vi "Move XYZ.vi"(0 "PID Gains In":T2={"X PID"={"proportional gain (Kc)"=0.03, "integral time (Ti, min)"=0.0, "derivative time (Td, min)"=0.0}, "Y PID"={"proportional gain (Kc)"=0.03, "integral time (Ti, min)"=0.0, "derivative time (Td, min)"=0.0}, "Z PID"={"proportional gain (Kc)"=0.035, "integral time (Ti, min)"=0.0, "derivative time (Td, min)"=0.0}} {"Z PID"."derivative time (Td, min)" format="%.3f"; "Z PID"."integral time (Ti, min)" format="%.3f"; "Z PID"."proportional gain (Kc)" format="%.3f"; "Y PID"."derivative time (Td, min)" format="%.3f"; "Y PID"."integral time (Ti, min)" format="%.3f"; "Y PID"."proportional gain (Kc)" format="%.3f"; "X PID"."derivative time (Td, min)" format="%.3f"; "X PID"."integral time (Ti, min)" format="%.3f"; "X PID"."proportional gain (Kc)" format="%.3f"}, 5 "Y Target":dbl, 6 "X Target":dbl, 10 "Max Time":dbl=90.0, 11 "Gyro Target":dbl=-180.0, 12 "Movement":dbl=3.0, 14 "X Output Range":cluster{"output high":dbl, "output low":dbl}={"output high"=0.8, "output low"=-0.8}, 15 "X Stop Threshold":dbl=5.0, 16 "Y Output Range":cluster{"output high":dbl, "output low":dbl}={"output high"=0.8, "output low"=-0.8}, 17 "Y Stop Threshold":dbl=5.0, 18 "Z Output Range":cluster{"output high":dbl, "output low":dbl}={"output high"=0.8, "output low"=-0.8}, 19 "Z  Stop Threshold":dbl=8.0) -> ()   [LabVIEW 2018]
uses:
  Robot Global Data.vi
  SubSystems/Drive Train/Drive Train Global.vi
  SubSystems/Hatch Panel Intake/Hatch Panel Intake Global.vi
  SubSystems/Lift/Lift Global.vi
  <vilib>/addons/control/pid/pid.llb/PID (DBL).vi
  <vilib>/addons/control/pid/NI_PID_pid.lvlib
panel:
  in  "Camera Tracking":T1={"proportional gain (Kc)"=0.06, "integral time (Ti, min)"=0.0, "derivative time (Td, min)"=0.0}
  in  "Minimum Time":u32=500
  in  "Settle Time":u32=2000
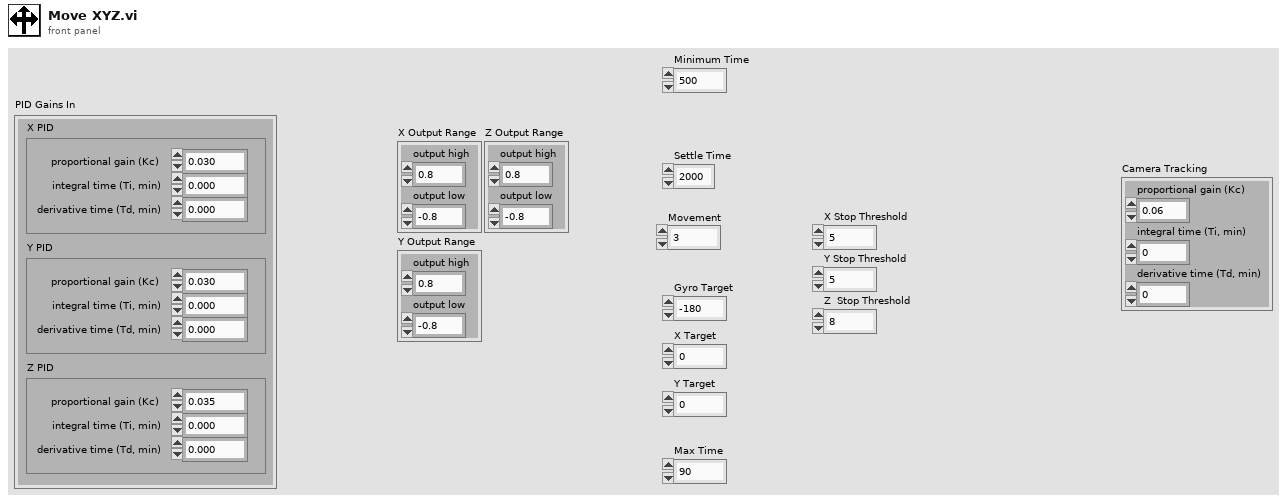
[diagram p1: front panel]
types:
  T1 = cluster{"proportional gain (Kc)":dbl, "integral time (Ti, min)":dbl, "derivative time (Td, min)":dbl}
  T2 = cluster{"X PID":cluster{"proportional gain (Kc)":dbl, "integral time (Ti, min)":dbl, "derivative time (Td, min)":dbl}, "Y PID":cluster{"proportional gain (Kc)":dbl, "integral time (Ti, min)":dbl, "derivative time (Td, min)":dbl}, "Z PID":cluster{"proportional gain (Kc)":dbl, "integral time (Ti, min)":dbl, "derivative time (Td, min)":dbl}}
  T3 = cluster{"Rollover":dbl, "Yaw":dbl, "Cont Yaw":dbl}
  T4 = cluster{"offsetAngle H":dbl, "offsetAngle V":dbl, "area":dbl, "skew":dbl, "validTarget":dbl, "latency":dbl}
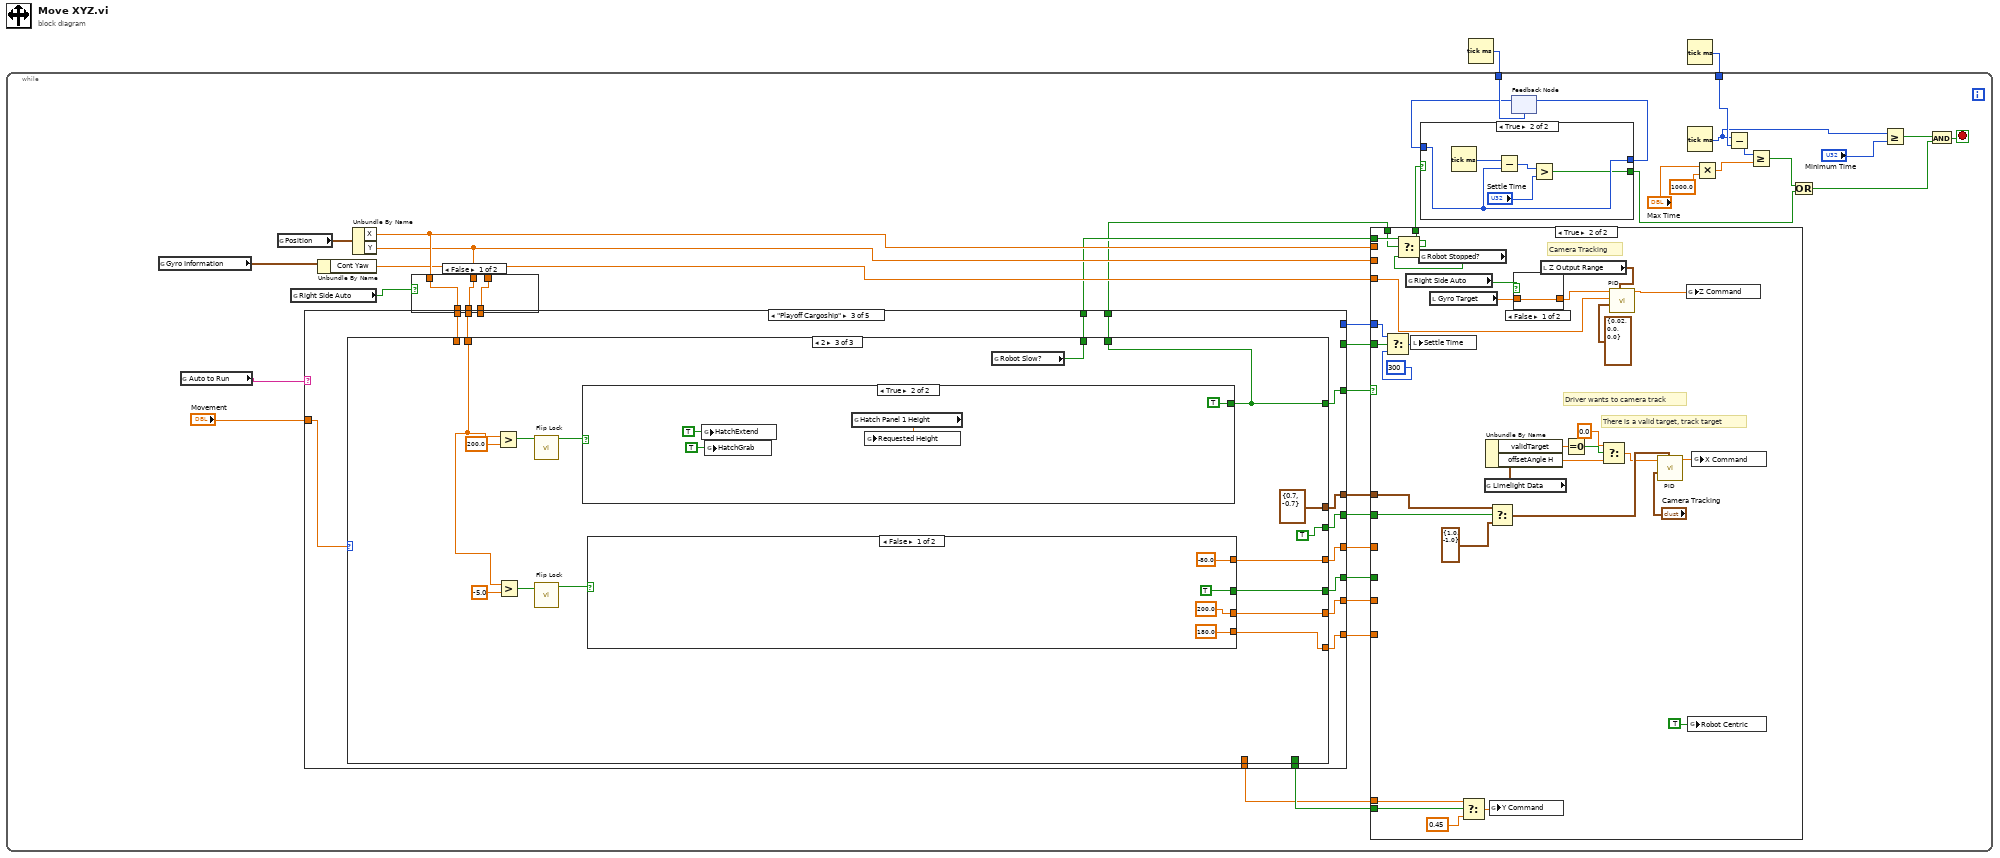
[diagram p0: block diagram]
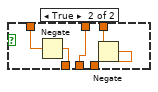
[diagram p2: hidden frame]
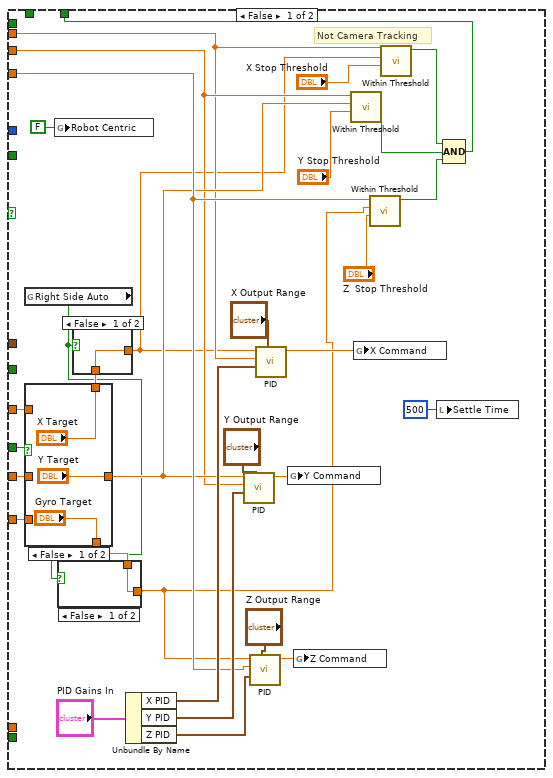
[diagram p3: hidden frame]
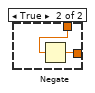
[diagram p4: hidden frame]
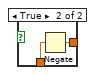
[diagram p5: hidden frame]
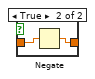
[diagram p7: hidden frame]
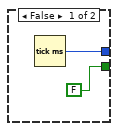
[diagram p8: hidden frame]
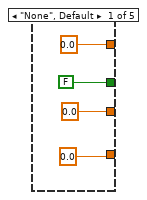
[diagram p9: hidden frame]
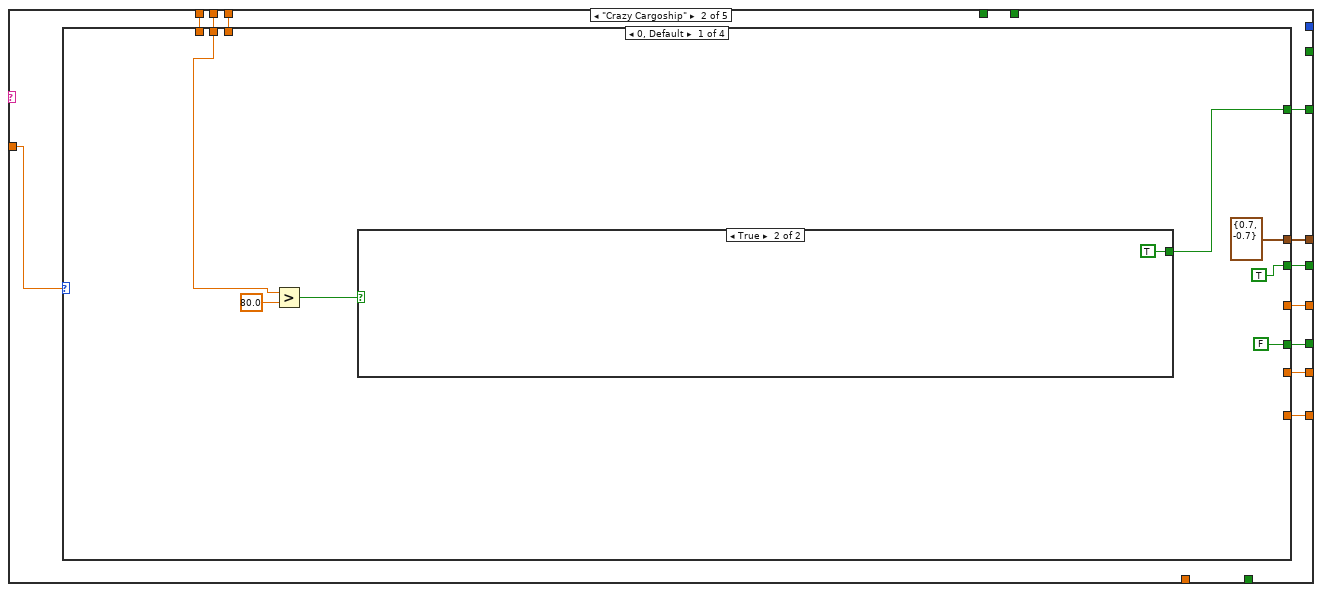
[diagram p10: hidden frame]
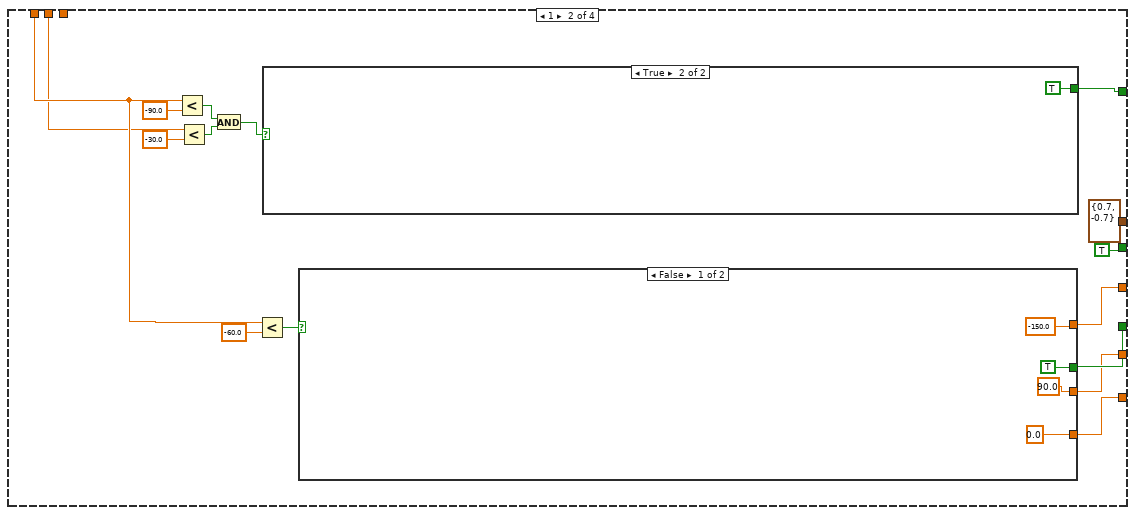
[diagram p12: hidden frame]
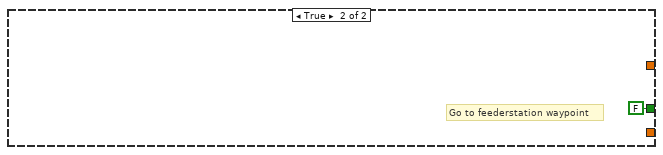
[diagram p13: hidden frame]
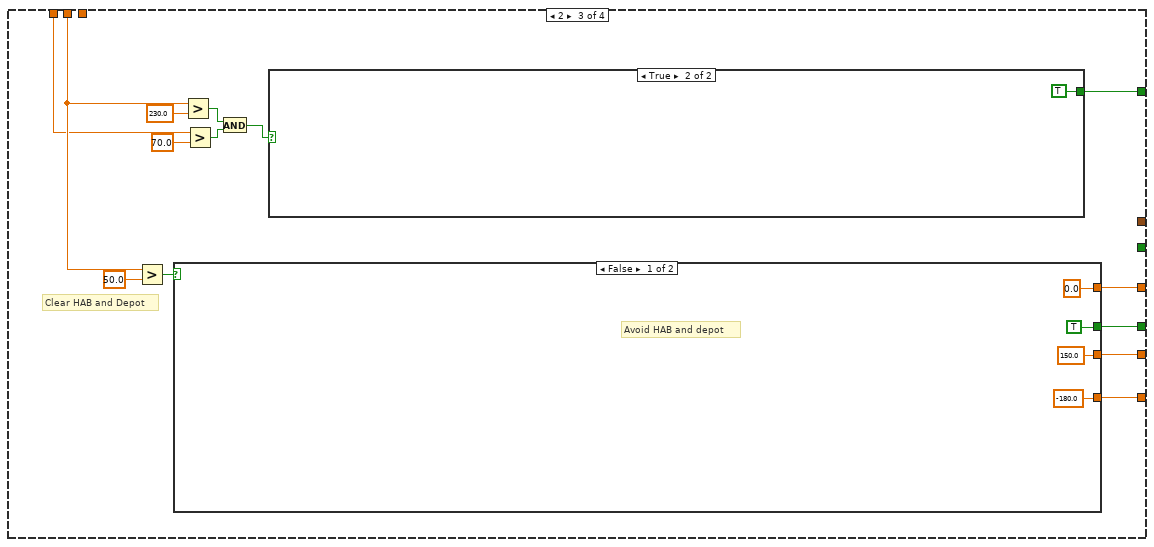
[diagram p15: hidden frame]
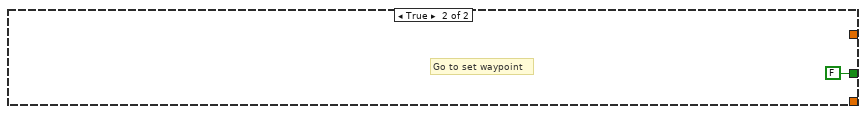
[diagram p17: hidden frame]
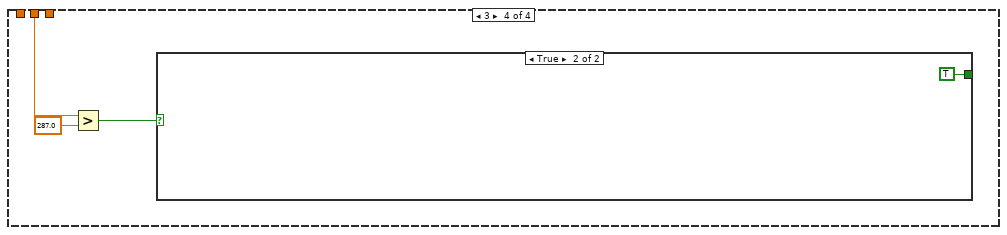
[diagram p18: hidden frame]
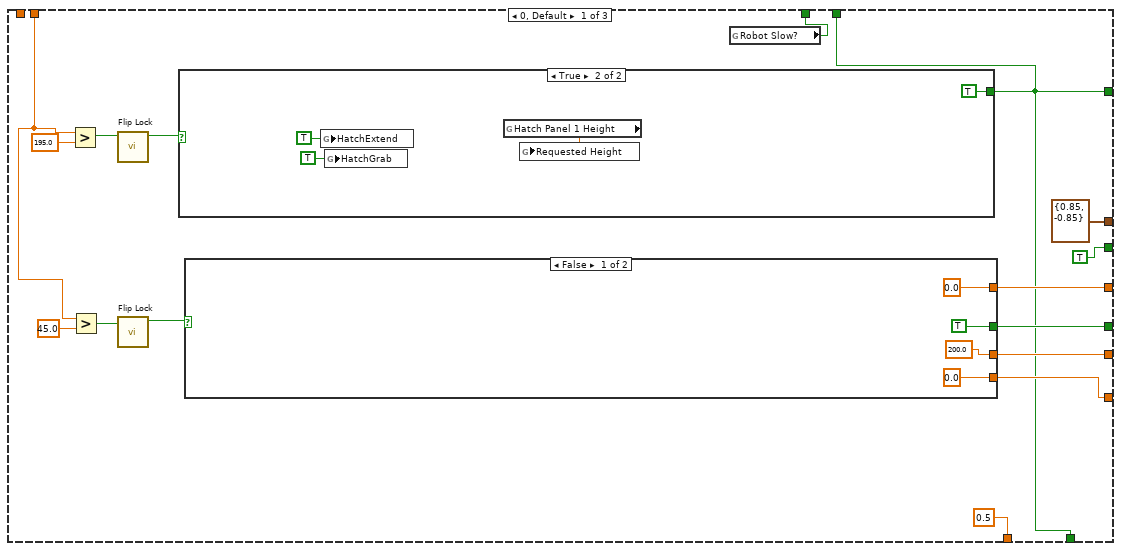
[diagram p20: hidden frame]
diagram:
  n1 = Tick Count (ms)() -> (millisecond timer value=w2:u32)
  n2 = Tick Count (ms)() -> (millisecond timer value=w1:u32)
  n3 = while {
    tunnel: w2 -> [w36]
    tunnel: w1 -> [w24]
    stop <- w23 stop-if-true
    n4 = global read "Drive Train Global.vi" "Gyro Information"() -> (w30:T3)
    n5 = global read "Robot Global Data.vi" "Auto to Run"() -> (w33:string)
    n6 = global read "Drive Train Global.vi" "Position"() -> (w32:cluster{"X":dbl, "Y":dbl})
    n7 = global read "Robot Global Data.vi" "Right Side Auto"() -> (w7:bool)
    n8 = Unbundle By Name(w30) -> ("Cont Yaw"=w9:dbl)
    n9 = Unbundle By Name(w32) -> ("X"=w12:dbl, "Y"=w10:dbl)
    n10 = case shown="False" w7 {
      tunnel: [w45 w50] -> w13
      tunnel: w12 -> [w45 w49]
      tunnel: [w44 w48] -> w11
      tunnel: w10 -> [w44 w48]
      tunnel: w9 -> [w43 w47]
      tunnel: [w43 w46] -> w8
      frame False {
      }
      frame True {
        n11 = Negate(x=w49) -> (-x=w50:dbl)
        n12 = Negate(x=w47) -> (-x=w46:dbl)
      }
    }
    n13 = case shown="\"Playoff Cargoship\"" w33 {
      tunnel: [0.0 w146 w213 w299 w394] -> w42
      tunnel: [0.0 w145 w211 w298 w393] -> w41
      tunnel: [0.0 w144 w210 w297 w392] -> w40
      tunnel: w11 -> [_ w150 w218 w302 w397]
      tunnel: [FALSE w149 w212 w300 w395] -> w39
      tunnel: w13 -> [_ w147 w219 w301 w396]
      tunnel: "Movement" -> [_ w151 w217 w303 w398]
      tunnel: w8 -> [_ w148 _ _ w390]
      tunnel: [_ w143 w215 w296 w391] -> w18
      tunnel: [_ w141 w216 w294 _] -> w17
      tunnel: [_ w142 w214 w295 _] -> w16
      tunnel: [_ _ _ w293 w389] -> w15
      tunnel: [_ _ _ w292 w388] -> w14
      tunnel: [_ _ w207 w291 _] -> w6
      tunnel: [_ _ w206 w290 _] -> w5
      tunnel: [_ _ w208 w289 _] -> w4
      tunnel: [_ _ w209 w288 _] -> w3
      frame "None", Default {
      }
      frame "Crazy Cargoship" {
        n14 = case shown="0, Default" w151 {
          tunnel: w150 -> [w154 w164 w183 w202]
          tunnel: [FALSE w175 w195 _] -> w149
          tunnel: w148 -> [_ _ _ _]
          tunnel: w147 -> [_ w165 w182 _]
          tunnel: [_ w174 w192 _] -> w146
          tunnel: [_ w173 w191 _] -> w145
          tunnel: [_ w172 w190 _] -> w144
          tunnel: [w156 w166 w184 _] -> w143
          tunnel: [TRUE ("Robot Centric") TRUE ("Robot Centric") _ _] -> w142
          tunnel: [cluster{"output high":dbl, "output low":dbl} {"output high"=0.7, "output low"=-0.7} ("output range") cluster{"output high":dbl, "output low":dbl} {"output high"=0.7, "output low"=-0.7} ("output range") _ _] -> w141
          frame 0, Default {
            n15 = Greater?(x=w154, y=80.0) -> (0:w155:bool)
            n16 = case shown="True" w155 {
              tunnel: [_ TRUE] -> w156
              frame False {
              }
              frame True {
              }
            }
          }
          frame 1 {
            n17 = Less?(x=w165, y=-90.0) -> (x < y?=w169:bool)
            n18 = Less?(x=w164, y=-30.0) -> (x < y?=w168:bool)
            n19 = And(x=w169, y=w168) -> (x .and. y?=w167:bool)
            n20 = Less?(x=w165, y=-60.0) -> (x < y?=w160:bool)
            n21 = case shown="True" w167 {
              tunnel: [_ TRUE] -> w166
              frame False {
              }
              frame True {
              }
            }
            n22 = case shown="False" w160 {
              tunnel: [TRUE FALSE] -> w175
              tunnel: [-150.0 _] -> w174
              tunnel: [90.0 _] -> w173
              tunnel: [0.0 _] -> w172
              frame False {
              }
              frame True {
                # "Go to feederstation waypoint"
              }
            }
          }
          frame 2 {
            # "Clear HAB and Depot"
            n23 = Greater?(x=w183, y=50.0) -> (0:w194:bool)
            n24 = case shown="False" w194 {
              tunnel: [TRUE FALSE] -> w195
              tunnel: [0.0 _] -> w192
              tunnel: [150.0 _] -> w191
              tunnel: [-180.0 _] -> w190
              frame False {
                # "Avoid HAB and depot"
              }
              frame True {
                # "Go to set waypoint"
              }
            }
            n25 = Greater?(x=w183, y=230.0) -> (0:w187:bool)
            n26 = Greater?(x=w182, y=70.0) -> (0:w186:bool)
            n27 = And(x=w187, y=w186) -> (x .and. y?=w185:bool)
            n28 = case shown="True" w185 {
              tunnel: [_ TRUE] -> w184
              frame False {
              }
              frame True {
              }
            }
          }
          frame 3 {
            n29 = Greater?(x=w202, y=287.0) -> (0:w203:bool)
            n30 = case shown="True" w203 {
              tunnel: [_ TRUE] -> _
              frame False {
              }
              frame True {
              }
            }
          }
        }
      }
      frame "Playoff Cargoship" {
        n31 = case shown="2" w217 {
          tunnel: w218 -> [w231 w246 w275]
          tunnel: [w229 w249 w273] -> w212
          tunnel: w219 -> [_ _ _]
          tunnel: [w230 w250 w274] -> w213
          tunnel: [w228 w248 w272] -> w211
          tunnel: [w227 w247 w271] -> w210
          tunnel: [w220 w244 w266] -> w215
          tunnel: [TRUE ("Robot Centric") _ TRUE ("Robot Centric")] -> w214
          tunnel: [cluster{"output high":dbl, "output low":dbl} {"output high"=0.85, "output low"=-0.85} ("output range") _ cluster{"output high":dbl, "output low":dbl} {"output high"=0.7, "output low"=-0.7} ("output range")] -> w216
          tunnel: [w220 w244 w266] -> w209
          tunnel: [w221 w245 w265] -> w208
          tunnel: [w220 _ _] -> w207
          tunnel: [0.5 ("Y Command") _ _] -> w206
          frame 0, Default {
            n32 = Greater?(x=w231, y=195.0) -> (0:w224:bool)
            n33 = Greater?(x=w231, y=45.0) -> (0:w226:bool)
            n34 = call "Flip Lock.vi"("Input"=w224) -> ("Output"=w223:bool)  [unwired: 10 in]
            n35 = call "Flip Lock.vi"("Input"=w226) -> ("Output"=w225:bool)  [unwired: 10 in]
            n36 = case shown="True" w223 {
              tunnel: [_ TRUE] -> w220
              frame False {
              }
              frame True {
                n37 = global write "Hatch Panel Intake Global.vi" "HatchExtend"(TRUE ("HatchExtend")) -> ()
                n38 = global write "Hatch Panel Intake Global.vi" "HatchGrab"(TRUE ("HatchGrab")) -> ()
                n39 = global read "Lift Global.vi" "Hatch Panel 1 Height"() -> (w242:dbl)
                n40 = global write "Lift Global.vi" "Requested Height"(w242) -> ()
              }
            }
            n41 = case shown="False" w225 {
              tunnel: [0.0 _] -> w230
              tunnel: [TRUE ("Robot Centric") _] -> w229
              tunnel: [200.0 _] -> w228
              tunnel: [0.0 _] -> w227
              frame False {
              }
              frame True {
              }
            }
            n42 = global read "Drive Train Global.vi" "Robot Slow?"() -> (w221:bool)
          }
          frame 1 {
            n43 = Less?(x=w246, y=45.0) -> (x < y?=w252:bool)
            n44 = Less?(x=w246, y=10.0) -> (x < y?=w255:bool)
            n45 = call "Flip Lock.vi"("Input"=w252) -> ("Output"=w251:bool)  [unwired: 10 in]
            n46 = call "Flip Lock.vi"("Input"=w255) -> ("Output"=w254:bool)  [unwired: 10 in]
            n47 = case shown="True" w254 {
              tunnel: [_ TRUE] -> w244
              frame False {
              }
              frame True {
                n48 = global write "Hatch Panel Intake Global.vi" "HatchExtend"(TRUE ("HatchExtend")) -> ()
                n49 = global write "Hatch Panel Intake Global.vi" "HatchGrab"(FALSE ("HatchGrab")) -> ()
                n50 = global read "Lift Global.vi" "Hatch Panel 1 Height"() -> (w263:dbl)
                n51 = global write "Lift Global.vi" "Requested Height"(w263) -> ()
              }
            }
            n52 = case shown="False" w251 {
              tunnel: [-85.0 _] -> w250
              tunnel: [TRUE ("Robot Centric") _] -> w249
              tunnel: [-100.0 _] -> w248
              tunnel: [180.0 _] -> w247
              frame False {
              }
              frame True {
              }
            }
            n53 = global read "Drive Train Global.vi" "Robot Slow?"() -> (w245:bool)
          }
          frame 2 {
            n54 = Greater?(x=w275, y=200.0) -> (0:w268:bool)
            n55 = Greater?(x=w275, y=-5.0) -> (0:w270:bool)
            n56 = call "Flip Lock.vi"("Input"=w268) -> ("Output"=w267:bool)  [unwired: 10 in]
            n57 = call "Flip Lock.vi"("Input"=w270) -> ("Output"=w269:bool)  [unwired: 10 in]
            n58 = case shown="True" w267 {
              tunnel: [_ TRUE] -> w266
              frame False {
              }
              frame True {
                n59 = global write "Hatch Panel Intake Global.vi" "HatchExtend"(TRUE ("HatchExtend")) -> ()
                n60 = global write "Hatch Panel Intake Global.vi" "HatchGrab"(TRUE ("HatchGrab")) -> ()
                n61 = global read "Lift Global.vi" "Hatch Panel 1 Height"() -> (w286:dbl)
                n62 = global write "Lift Global.vi" "Requested Height"(w286) -> ()
              }
            }
            n63 = case shown="False" w269 {
              tunnel: [-80.0 _] -> w274
              tunnel: [TRUE ("Robot Centric") _] -> w273
              tunnel: [200.0 _] -> w272
              tunnel: [180.0 _] -> w271
              frame False {
              }
              frame True {
              }
            }
            n64 = global read "Drive Train Global.vi" "Robot Slow?"() -> (w265:bool)
          }
        }
      }
      frame "Fun Rocket Close" {
        n65 = case shown="2" w303 {
          tunnel: w302 -> [w314 w334 w353 w376]
          tunnel: w301 -> [w315 w335 _ _]
          tunnel: [w319 _ w351 w371] -> w300
          tunnel: [w318 _ w352 w374] -> w299
          tunnel: [w317 _ w350 w373] -> w298
          tunnel: [w316 _ w349 w372] -> w297
          tunnel: [w307 w332 w348 w379] -> w296
          tunnel: [_ _ w357 _] -> w295
          tunnel: [_ _ w356 _] -> w294
          tunnel: [w307 w332 w348 _] -> w293
          tunnel: [u32 150 ("Settle Time") u32 150 ("Settle Time") u32 150 ("Settle Time") _] -> w292
          tunnel: [w307 TRUE _ _] -> w291
          tunnel: [0.6 ("Y Command") 0.55 ("Y Command") _ _] -> w290
          tunnel: [w305 w328 w345 w369] -> w289
          tunnel: [TRUE TRUE TRUE TRUE] -> w288
          frame 0, Default {
            # "Wait until robot gets off hab"
            n66 = Less?(x=w315, y=-45.0) -> (x < y?=w321:bool)
            n67 = Less?(x=w315, y=-70.0) -> (x < y?=w311:bool)
            n68 = Greater?(x=w314, y=50.0) -> (0:w310:bool)
            n69 = case shown="False" w321 {
              tunnel: [TRUE FALSE] -> w319
              tunnel: [-120.0 _] -> w318
              tunnel: [0.0 _] -> w317
              tunnel: [0.0 _] -> w316
              frame False {
                # "Go straight to the right off of the HAB"
              }
              frame True {
                # "Robot off of HAB, go to the rocket"
              }
            }
            n70 = And(x=w311, y=w310) -> (x .and. y?=w309:bool)
            n71 = case shown="True" w309 {
              tunnel: [_ TRUE] -> w307
              frame False {
              }
              frame True {
              }
            }
            n72 = global read "Drive Train Global.vi" "Robot Slow?"() -> (w305:bool)
          }
          frame 1 {
            n73 = Less?(x=w334, y=25.0) -> (x < y?=w338:bool)
            n74 = Less?(x=w335, y=10.0) -> (x < y?=w337:bool)
            n75 = And(x=w338, y=w337) -> (x .and. y?=w336:bool)
            n76 = case shown="True" w336 {
              tunnel: [_ TRUE] -> w332
              frame False {
              }
              frame True {
                n77 = global write "Hatch Panel Intake Global.vi" "HatchExtend"(TRUE ("HatchExtend")) -> ()
                n78 = global write "Hatch Panel Intake Global.vi" "HatchGrab"(FALSE ("HatchGrab")) -> ()
                n79 = global read "Lift Global.vi" "Hatch Panel 1 Height"() -> (w341:dbl)
                n80 = global write "Lift Global.vi" "Requested Height"(w341) -> ()
              }
            }
            n81 = global read "Drive Train Global.vi" "Robot Slow?"() -> (w328:bool)
          }
          frame 2 {
            # "back up then turn"
            n82 = Greater?(x=w353, y=160.0) -> (0:w358:bool)
            n83 = Greater?(x=w353, y=40.0) -> (0:w354:bool)
            n84 = case shown="True" w358 {
              tunnel: [_ TRUE] -> w348
              tunnel: [_ TRUE] -> w357
              tunnel: [_ cluster{"output high":dbl, "output low":dbl} {"output high"=0.6, "output low"=-0.6} ("output range")] -> w356
              frame False {
              }
              frame True {
                n85 = global read "Lift Global.vi" "Hatch Panel 1 Height"() -> (w365:dbl)
                n86 = global write "Lift Global.vi" "Requested Height"(w365) -> ()
              }
            }
            n87 = case shown="False" w354 {
              tunnel: [0.0 _] -> w352
              tunnel: [TRUE FALSE] -> w351
              tunnel: [200.0 _] -> w350
              tunnel: [-180.0 _] -> w349
              frame False {
              }
              frame True {
              }
            }
            n88 = global read "Drive Train Global.vi" "Robot Slow?"() -> (w345:bool)
          }
          frame 3 {
            n89 = Less?(x=w376, y=30.0) -> (x < y?=w378:bool)
            n90 = Less?(x=w376, y=140.0) -> (x < y?=w375:bool)
            n91 = case shown="True" w375 {
              tunnel: [0.0 _] -> w374
              tunnel: [100.0 _] -> w373
              tunnel: [-30.0 _] -> w372
              tunnel: [TRUE _] -> w371
              frame False {
              }
              frame True {
              }
            }
            n92 = case shown="True" w378 {
              tunnel: [_ TRUE] -> w379
              frame False {
              }
              frame True {
                n93 = global write "Hatch Panel Intake Global.vi" "HatchExtend"(TRUE ("HatchGrab")) -> ()
                n94 = global write "Hatch Panel Intake Global.vi" "HatchGrab"(FALSE ("HatchGrab")) -> ()
              }
            }
            n95 = global read "Drive Train Global.vi" "Robot Slow?"() -> (w369:bool)
          }
        }
      }
      frame "Fun Rocket Far" {
        n96 = case shown="1" w398 {
          tunnel: w397 -> [w404 w434 w469 w485]
          tunnel: w396 -> [w403 w441 _ _]
          tunnel: [w409 w439 w474 w480] -> w395
          tunnel: [w408 w440 w473 w483] -> w394
          tunnel: [w407 w438 w472 w482] -> w393
          tunnel: [w406 w437 w471 w481] -> w392
          tunnel: [w405 w443 _ w488] -> w391
          tunnel: w390 -> [_ _ _ _]
          tunnel: [w401 _ _ _] -> w389
          tunnel: [w402 _ _ _] -> w388
          frame 0, Default {
            # "Move to far rocket"
            # "Wait until robot gets off hab"
            n97 = Greater?(x=w404, y=210.0) -> (0:w399:bool)
            n98 = call "Flip Lock.vi"("Input"=w399) -> ("Output"=w400:bool)  [unwired: 10 in]
            n99 = case shown="True" w400 {
              tunnel: [TRUE w425] -> w409
              tunnel: [-10.0 w424] -> w408
              tunnel: [250.0 w423] -> w407
              tunnel: [0.0 w422] -> w406
              tunnel: [_ w421] -> w405
              tunnel: w403 -> [_ w419]
              tunnel: [_ w416] -> w402
              tunnel: [_ w415] -> w401
              frame False {
              }
              frame True {
                # "Wait for robot to be in good\nplace to camera track"
                n100 = Less?(x=w419, y=-80.0) -> (x < y?=w418:bool)
                n101 = call "Flip Lock.vi"("Input"=w418) -> ("Output"=w417:bool)  [unwired: 10 in]
                n102 = case shown="False" w417 {
                  tunnel: [TRUE FALSE] -> w425
                  tunnel: [-150.0 ("y") _] -> w424
                  tunnel: [230.0 ("y") _] -> w423
                  tunnel: [-130.0 ("y") _] -> w422
                  tunnel: [FALSE w431] -> w421
                  tunnel: [_ u32 500 ("Settle Time")] -> w416
                  tunnel: [_ w431] -> w415
                  frame False {
                  }
                  frame True {
                    w431 = TRUE
                  }
                }
              }
            }
          }
          frame 1 {
            n103 = Less?(x=w434, y=-30.0) -> (x < y?=w446:bool)
            n104 = Less?(x=w441, y=0.0) -> (x < y?=w445:bool)
            n105 = And(x=w446, y=w445) -> (x .and. y?=w444:bool)
            n106 = Greater?(x=w441, y=-60.0) -> (0:w435:bool)
            n107 = case shown="False" w444 {
              tunnel: [FALSE TRUE] -> w443
              frame False {
              }
              frame True {
              }
            }
            n108 = call "Flip Lock.vi"("Input"=w435) -> ("Output"=w436:bool)  [unwired: 10 in]
            n109 = case shown="True" w436 {
              tunnel: [0.0 ("y") w455] -> w440
              tunnel: [TRUE w456] -> w439
              tunnel: [230.0 ("y") w454] -> w438
              tunnel: [-150.0 ("y") w453] -> w437
              tunnel: w434 -> [_ w458]
              frame False {
              }
              frame True {
                n110 = Less?(x=w458, y=40.0) -> (x < y?=w459:bool)
                n111 = call "Flip Lock.vi"("Input"=w459) -> ("Output"=w460:bool)  [unwired: 10 in]
                n112 = case shown="True" w460 {
                  tunnel: [TRUE FALSE] -> w456
                  tunnel: [-70.0 ("y") _] -> w455
                  tunnel: [-40.0 ("y") _] -> w454
                  tunnel: [-180.0 ("y") _] -> w453
                  frame False {
                  }
                  frame True {
                  }
                }
              }
            }
          }
          frame 2 {
            n113 = Less?(x=w469, y=30.0) -> (x < y?=w470:bool)
            n114 = case shown="False" w470 {
              tunnel: [TRUE FALSE] -> w474
              tunnel: [-30.0 _] -> w473
              tunnel: [100.0 _] -> w472
              tunnel: [-180.0 _] -> w471
              frame False {
              }
              frame True {
              }
            }
          }
          frame 3 {
            n115 = Less?(x=w485, y=30.0) -> (x < y?=w487:bool)
            n116 = Less?(x=w485, y=140.0) -> (x < y?=w484:bool)
            n117 = case shown="False" w484 {
              tunnel: [0.0 _] -> w483
              tunnel: [100.0 _] -> w482
              tunnel: [-30.0 _] -> w481
              tunnel: [TRUE _] -> w480
              frame False {
              }
              frame True {
              }
            }
            n118 = case shown="True" w487 {
              tunnel: [_ TRUE] -> w488
              frame False {
              }
              frame True {
              }
            }
          }
        }
      }
    }
    n119 = case shown="True" w18 {
      tunnel: w42 -> [w75 _]
      tunnel: w41 -> [w74 _]
      tunnel: w40 -> [w73 _]
      tunnel: w39 -> [w72 _]
      tunnel: [w58 w98] -> w29
      tunnel: w9 -> [w67 w122]
      tunnel: w10 -> [w63 _]
      tunnel: w12 -> [w60 _]
      tunnel: w17 -> [_ w118]
      tunnel: w16 -> [_ w117]
      tunnel: w15 -> [_ w114]
      tunnel: w14 -> [_ w113]
      tunnel: w6 -> [_ w101]
      tunnel: w5 -> [_ w100]
      tunnel: w4 -> [_ w97]
      tunnel: w3 -> [_ w96]
      frame False {
        # "Not Camera Tracking"
        n120 = global read "Robot Global Data.vi" "Right Side Auto"() -> (w51:bool)
        n121 = case shown="False" w72 {
          tunnel: ["X Target" w94] -> w55
          tunnel: ["Y Target" w93] -> w64
          tunnel: ["Gyro Target" w92] -> w53
          tunnel: w75 -> [_ w94]
          tunnel: w74 -> [_ w93]
          tunnel: w73 -> [_ w92]
          frame False {
          }
          frame True {
          }
        }
        n122 = global write "Drive Train Global.vi" "Robot Centric"(FALSE ("Robot Centric")) -> ()
        n123 = case shown="False" w51 {
          tunnel: w53 -> [w83 w84]
          tunnel: [w83 w85] -> w52
          frame False {
          }
          frame True {
            n124 = Negate(x=w84) -> (-x=w85:dbl)
          }
        }
        n125 = case shown="False" w51 {
          tunnel: w55 -> [w86 w87]
          tunnel: [w86 w88] -> w54
          frame False {
          }
          frame True {
            n126 = Negate(x=w87) -> (-x=w88:dbl)
          }
        }
        n127 = Unbundle By Name("PID Gains In") -> ("X PID"=w80:T1, "Y PID"=w79:T1, "Z PID"=w78:T1)
        n128 = call-poly <vilib>:"PID.vi"("output range"="Y Output Range", "PID gains"=w79, "process variable"=w63, "setpoint"=w64) -> ("output"=w69:dbl)  [unwired: 6 in, 1 out]
        n129 = call-poly <vilib>:"PID.vi"("output range"="Z Output Range", "PID gains"=w78, "process variable"=w67, "setpoint"=w52) -> ("output"=w70:dbl)  [unwired: 6 in, 1 out]
        n130 = call-poly <vilib>:"PID.vi"("output range"="X Output Range", "PID gains"=w80, "process variable"=w60, "setpoint"=w54) -> ("output"=w71:dbl)  [unwired: 6 in, 1 out]
        n131 = global write "Drive Train Global.vi" "Y Command"(w69) -> ()
        n132 = global write "Drive Train Global.vi" "Z Command"(w70) -> ()
        n133 = call "Within Threshold.vi"("Threshold"="Y Stop Threshold", "Center"=w64, "Value"=w63) -> ("Within Threshold?"=w65:bool)  [unwired: 8 in]
        n134 = global write "Drive Train Global.vi" "X Command"(w71) -> ()
        n135 = call "Within Threshold.vi"("Threshold"="Z  Stop Threshold", "Center"=w52, "Value"=w67) -> ("Within Threshold?"=w68:bool)  [unwired: 8 in]
        n136 = call "Within Threshold.vi"("Threshold"="X Stop Threshold", "Center"=w54, "Value"=w60) -> ("Within Threshold?"=w61:bool)  [unwired: 8 in]
        n137 = local write "Settle Time"(u32 500 ("Settle Time")) -> ()
        n138 = Compound Arithmetic op=AND(w61, w65, w68) -> (w58:bool)
      }
      frame True {
        # "There is a valid target, track target"
        # "Driver wants to camera track"
        # "Camera Tracking"
        n139 = Select(t=w113, s=w114, f=u32 300 ("Settle Time")) -> (s? t:f=w116:u32)
        n140 = global read "Robot Global Data.vi" "Right Side Auto"() -> (w105:bool)
        n141 = local write "Settle Time"(w116) -> ()
        n142 = global read "Drive Train Global.vi" "Robot Stopped?"() -> (w99:bool)
        n143 = Select(t=w97, s=w96, f=w99) -> (s? t:f=w98:bool)
        n144 = local read "Gyro Target"() -> (w107:dbl)
        n145 = Select(t=w100, s=w101, f=0.45 ("Y Command")) -> (s? t:f=w103:dbl)
        n146 = global read "Robot Global Data.vi" "Limelight Data"() -> (w125:T4)
        n147 = Unbundle By Name(w125) -> ("validTarget"=w112:dbl, "offsetAngle H"=w111:dbl)
        n148 = global write "Drive Train Global.vi" "Y Command"(w103) -> ()
        n149 = Select(t=w118, s=w117, f=cluster{"output high":dbl, "output low":dbl} {"output high"=1.0, "output low"=-1.0} ("output range")) -> (s? t:f=w119:cluster{"output high":dbl, "output low":dbl})
        n150 = case shown="False" w105 {
          tunnel: w107 -> [w127 w128]
          tunnel: [w127 w129] -> w106
          frame False {
          }
          frame True {
            n151 = Negate(x=w128) -> (-x=w129:dbl)
          }
        }
        n152 = local read "Z Output Range"() -> (w123:cluster{"output high":dbl, "output low":dbl})
        n153 = Equal To 0?(x=w112) -> (x = 0?=w109:bool)
        n154 = Select(t=0.0, s=w109, f=w111) -> (s? t:f=w110:dbl)
        n155 = call-poly <vilib>:"PID.vi"("output range"=w123, "PID gains"=T1 {"proportional gain (Kc)"=0.02, "integral time (Ti, min)"=0.0, "derivative time (Td, min)"=0.0}, "process variable"=w122, "setpoint"=w106) -> ("output"=w104:dbl)  [unwired: 6 in, 1 out]
        n156 = call-poly <vilib>:"PID.vi"("output range"=w119, "PID gains"="Camera Tracking", "setpoint"=w110) -> ("output"=w126:dbl)  [unwired: 7 in, 1 out]
        n157 = global write "Drive Train Global.vi" "Z Command"(w104) -> ()
        n158 = global write "Drive Train Global.vi" "Robot Centric"(TRUE ("Robot Centric")) -> ()
        n159 = global write "Drive Train Global.vi" "X Command"(w126) -> ()
      }
    }
    n160 = feedback #1(w36) -> (w35:u32)
    n161 = case shown="True" w29 {
      tunnel: [w131 w134] -> w37
      tunnel: w35 -> [_ w134]
      tunnel: [FALSE w133] -> w34
      frame False {
        n162 = Tick Count (ms)() -> (millisecond timer value=w131:u32)
      }
      frame True {
        n163 = Tick Count (ms)() -> (millisecond timer value=w136:u32)
        n164 = Subtract(x=w136, y=w134) -> (x-y=w135:u32)
        n165 = Greater?(x=w135, y="Settle Time") -> (0:w133:bool)
      }
    }
    n166 = feedback-in #1(w37) -> ()
    n167 = Tick Count (ms)() -> (millisecond timer value=w22:u32)
    n168 = Multiply(x="Max Time", y=1000.0) -> (x*y=w27:dbl)
    n169 = Subtract(x=w22, y=w24) -> (x-y=w28:u32)
    n170 = Greater Or Equal?(x=w28, y=w27) -> (x >= y?=w38:bool)
    n171 = Or(x=w38, y=w34) -> (x .or. y?=w19:bool)
    n172 = Greater Or Equal?(x=w22, y="Minimum Time") -> (x >= y?=w20:bool)
    n173 = And(x=w20, y=w19) -> (x .and. y?=w23:bool)
  }
